vi "RT Driver VI.vi"(7 "Operation":T1, 11 "Device Reference in":T2 format="%.0x") -> (0 "Error Code":i32)   [LabVIEW 2016, in "PXImc Custom Device Engine.lvlib"]
uses:
  PXImc Custom Device Engine.lvlib
  <vilib>/NI Veristand/Custom Device API/Custom Device Item Ref.ctl
  <vilib>/NI Veristand/Custom Device API/Hardware Interface Driver VI Operation.ctl
  Shared/Compiled.Settings.ctl
  PXImc Router/Controls/Target Type.ctl
  PXImc Router/Controls/Router - Configuration.ctl
  PXImc Router/Controls/Router/Node Block R-W Properties.ctl
  PXImc Router/Controls/Router/Block Properties.ctl
  PXImc Router/Controls/Router/Router - PXImc Properties.ctl
  PXImc Router/Controls/Router/Router - PXImc Card Properties.ctl
  PXImc Router/Controls/Node Data.ctl
  PXImc Router/Controls/Node/Node - PXImc Parameters.ctl
  PXImc Router/Controls/Node/Node - Writer Data.ctl
  PXImc Router/Controls/Node/Node Ch Properties.ctl
  PXImc Router/Controls/Data Type.ctl
  PXImc Router/Controls/Node/Node - Readers Data.ctl
  PXImc Router/Controls/Node/Node - Reader Data.ctl
  RTStateVariables.ctl
  <vilib>/NI/NIVS Inline Async API/_VS Inline Async API/VS Inline Async API/VS Inline Async API.lvclass
  <vilib>/NI/NIVS Inline Async API/_VS Inline Async API/VS Inline Async API/VS Inline Async API.lvclass/VS Inline Async API.ctl
  <vilib>/NI/NIVS Inline Async API/_Data Access Engine/Data Access Engine/Data Access Engine.lvclass/Data Access Engine.ctl
  <vilib>/NI/NIVS Inline Async API/_Data Access Engine/Access Type Classes/Write/Write.lvclass/Write.ctl
  <vilib>/NI/NIVS Inline Async API/_Data Access Engine/Access Type Classes/ReadWrite/ReadWrite.lvclass/ReadWrite.ctl
  <vilib>/NI/NIVS Inline Async API/_Data Access Engine/Access Type Classes/Read/Read.lvclass/Read.ctl
  <vilib>/NI/NIVS Inline Async API/_Data Access Engine/Data Access Engine/Methods/Data.Engine.Read Data from HW.vi
  <vilib>/NI/NIVS Inline Async API/_VS Inline Async API/Error Handling Process/SubVIs/Error.GetError.vi
  <vilib>/NI/NIVS Inline Async API/_Data Access Engine/Data Access Engine/Methods/Data.Engine.Write Data to HW.vi
  <vilib>/NI/NIVS Inline Async API/_Data Access Engine/Access Type Classes/ReadWrite/ReadWrite.EngineData.vi
  <vilib>/NI/NIVS Inline Async API/_Data Access Engine/Access Type Classes/Write/Write.EngineData.vi
  <vilib>/NI/NIVS Inline Async API/_Data Access Engine/Access Type Classes/Read/Read.EngineData.vi
  <vilib>/NI Veristand/Custom Device API/NI VeriStand - Get Channel Value by Data Reference.vi
  <vilib>/NI Veristand/Custom Device API/NI VeriStand - Set Channel Value by Data Reference.vi
  <vilib>/NI Veristand/Custom Device API/NI VeriStand - Get Channel Values by Block Data Reference.vi
  Shared/Constants.vi
  <vilib>/NI Veristand/Custom Device API/Get Item Property (Variant).vi
  <vilib>/NI Veristand/Custom Device API/Global Data Refs.vi
  <vilib>/NI VeriStand/Custom Device API/Custom Device API.lvlib
  <vilib>/NI VeriStand/Custom Device Tools/Custom Device Utility Library/Custom Device Utility Library.lvlib
  Shared/PXImc Custom Device Shared.lvlib
  PXImc Router/PXImc Router.lvlib
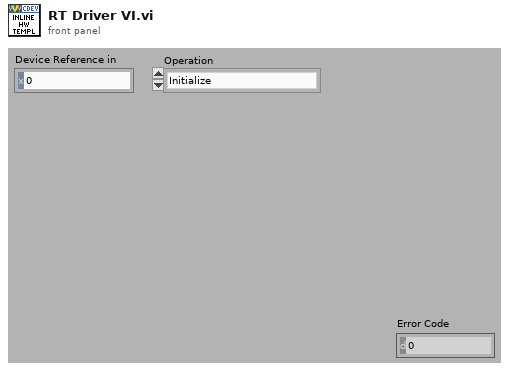
[diagram p1: front panel]
types:
  T1 = typedef "Custom Device API.lvlib/Hardware Interface Driver VI Operation.ctl" = enum16{"Initialize", "Start", "Read Data from HW", "Write Data to HW", "Close"}
  T2 = typedef "Custom Device API.lvlib/Custom Device Item Ref.ctl" = u64
  T3 = typedef "PXImc Custom Device Engine.lvlib/RTStateVariables.ctl" = cluster{"Async":refnum<class "VS Inline Async API.lvclass">, "Settings":T4}
  T4 = typedef "PXImc Custom Device Shared.lvlib/Compiled.Settings.ctl" = cluster{"Target Type":T5, "Router Properties":T6, "Node Data":T11, "Configuration Folder Path":path}
  T5 = typedef "PXImc Router.lvlib/Target Type.ctl" = enum16{"Router", "Node"}
  T6 = typedef "PXImc Router.lvlib/Router - Configuration.ctl" = cluster{"Target Type":T5, "Master Table Ref":refnum<data-value>, "Master Table Size (Bytes)":u32, "Node Properties":T7[], "Router - PXImc Properties":T9}
  T7 = typedef "PXImc Router.lvlib/Node Block R-W Properties.ctl" = cluster{"Node ID":u32, "# Reading Blocks":u32, "Node Writing Block":T8, "Node Reading Blocks":T8[]}
  T8 = typedef "PXImc Router.lvlib/Block Properties.ctl" = cluster{"Offset":u32, "Size (Bytes)":u32}
  T9 = typedef "PXImc Router.lvlib/Router - PXImc Properties.ctl" = cluster{"PXImc Cards Properties":T10[], "Connection Timeout (s)":dbl, "Readers Buffer Size":u64}
  T10 = typedef "PXImc Router.lvlib/Router - PXImc Card Properties.ctl" = cluster{"PXImc Resource Name":string, "Reader - PXImc Session Ref":refnum<k21>, "Writer - PXImc Session Ref":refnum<k21>, "Reader Conn ID":u16, "Writer Conn ID":u16}
  T11 = typedef "PXImc Router.lvlib/Node Data.ctl" = cluster{"Node Name":string, "PXImc Parameters":T12, "Local Data":T13, "Imported Data":T16}
  T12 = typedef "PXImc Router.lvlib/Node - PXImc Parameters.ctl" = cluster{"Resource Name":string, "Connection Timeout (s)":dbl, "Readers Buffer Size":u64, "Node PXImc Reader Conn Id":u16, "Node PXImc Writer Conn Id":u16, "Writer PXImc Session":refnum<k21>, "Reader PXImc Session":refnum<k21>}
  T13 = typedef "PXImc Router.lvlib/Node - Writer Data.ctl" = cluster{"Flattened Byte Buffer Ref":string, "Noder ID":u32, "Master Table Offest":u32, "Byte Buffer Size":u32, "Node Local Channels":T14[], "Node Local Channels Table":string[][]}
  T14 = typedef "PXImc Router.lvlib/Node Ch Properties.ctl" = cluster{"Name":string, "Value":dbl, "Data Type":T15}
  T15 = typedef "PXImc Router.lvlib/Data Type.ctl" = enum16{"Boolean", "SGL", "DBL", "I8", "I16", "I32", "I64", "U8", "U16", "U32", "U64"}
  T16 = typedef "PXImc Router.lvlib/Node - Readers Data.ctl" = cluster{"Flattened Byte Buffer Ref":string, "Byte Buffer Size":u64, "Readers Data Array":T17[], "Node Imported Channels Table":string[][]}
  T17 = typedef "PXImc Router.lvlib/Node - Reader Data.ctl" = cluster{"Noder ID":u32, "Master Table Offest":u32, "Byte Buffer Size":u64, "Node Imported Channels":T14[]}
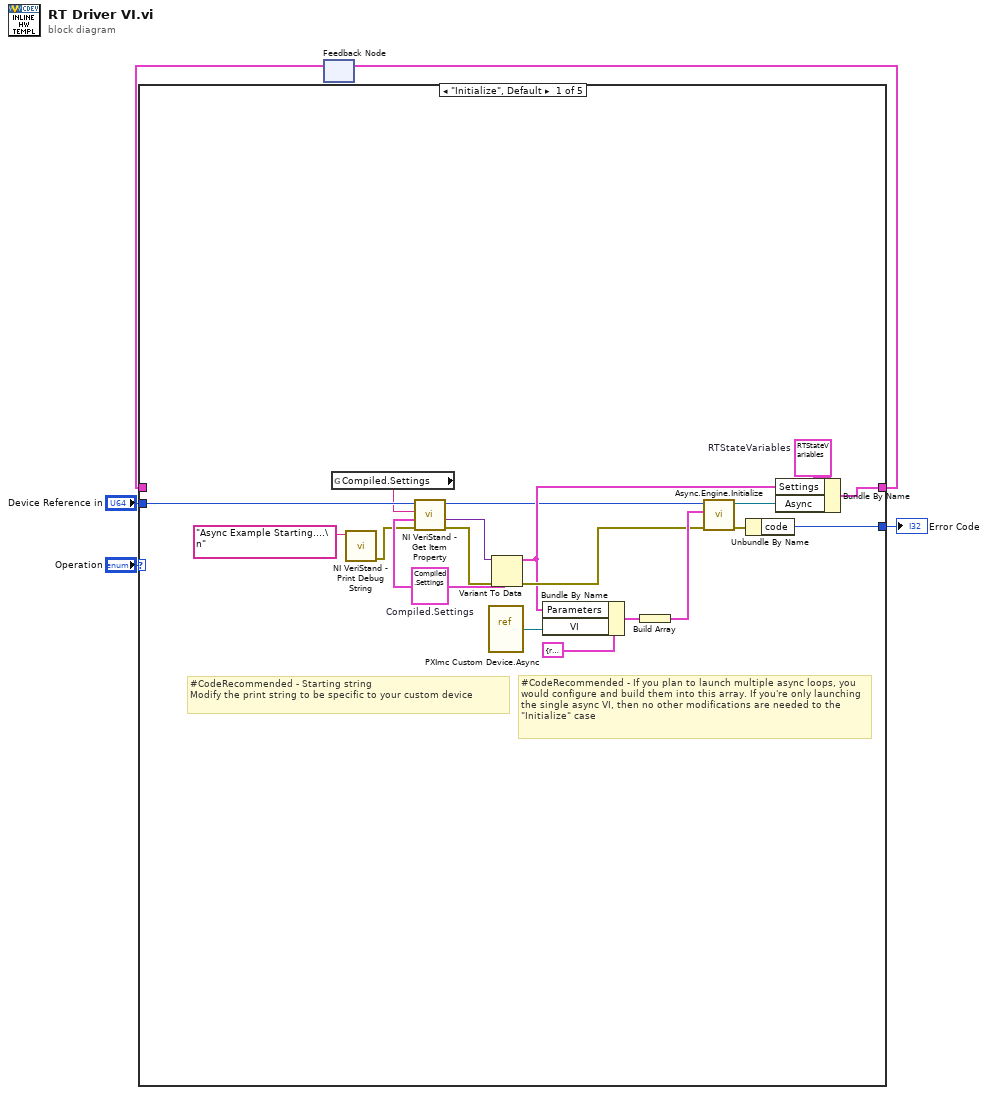
[diagram p0: block diagram]
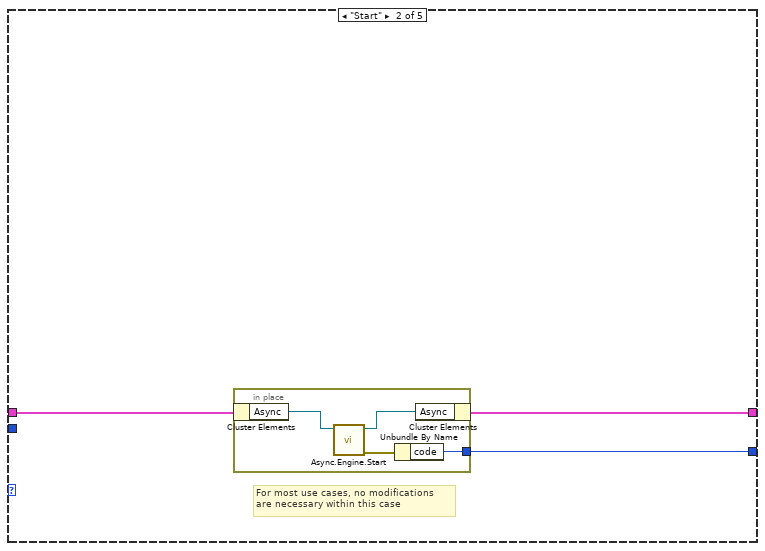
[diagram p2: hidden frame]
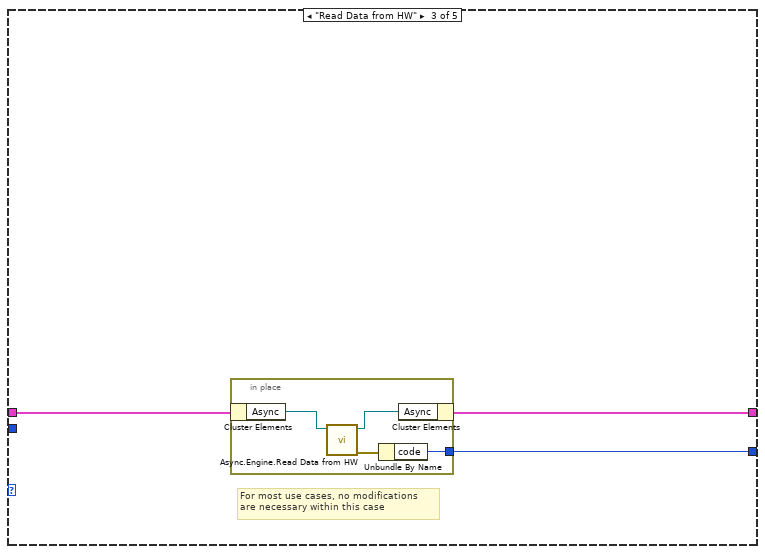
[diagram p3: hidden frame]
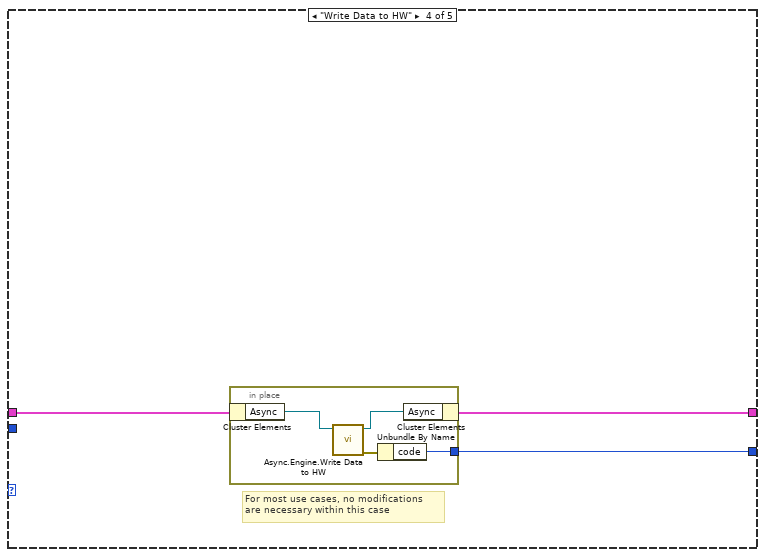
[diagram p4: hidden frame]
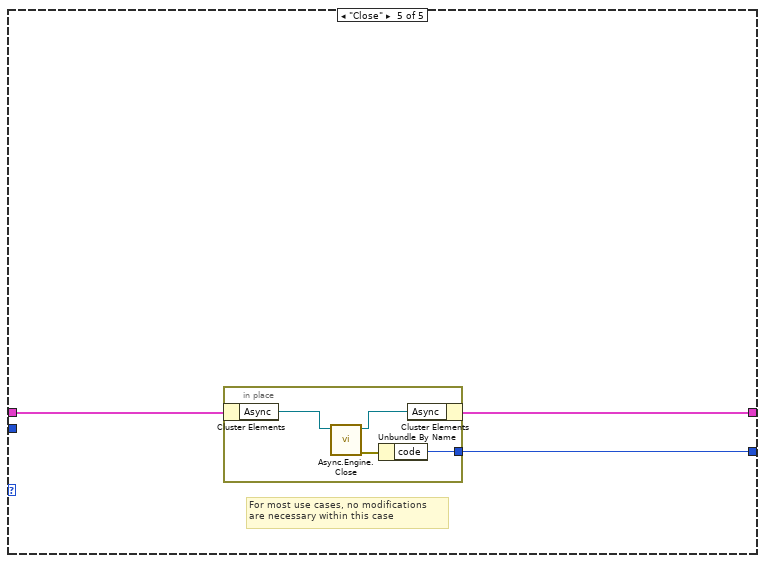
[diagram p5: hidden frame]
diagram:
  n1 = feedback #1() -> (w3:T3)  [unwired: 1 out]
  n2 = case shown="\"Initialize\", Default" "Operation" {
    tunnel: [w22 w26 w32 w39 w47] -> w4
    tunnel: w3 -> [_ w27 w34 w40 w48]
    tunnel: "Device Reference in" -> [w19 _ _ _ _]
    tunnel: [w24 w25 w33 w41 w46] -> w1
    frame "Initialize", Default {
      w15 = T3 {"Async"=refnum, "Settings"={"Target Type"=enum."Router", "Router Properties"={"Target Type"=enum."Router", "Master Table Ref"=refnum, "Master Table Size (Bytes)"=0, "Node Properties"=[], "Router - PXImc Properties"={"PXImc Cards Properties"=[], "Connection Timeout (s)"=0.0, "Readers Buffer Size"=0}}, "Node Data"={"Node Name"="", "PXImc Parameters"={"Resource Name"="", "Connection Timeout (s)"=0.0, "Readers Buffer Size"=0, "Node PXImc Reader Conn Id"=0, "Node PXImc Writer Conn Id"=0, "Writer PXImc Session"="", "Reader PXImc Session"=""}, "Local Data"={"Flattened Byte Buffer Ref"="", "Noder ID"=0, "Master Table Offest"=0, "Byte Buffer Size"=0, "Node Local Channels"=[], "Node Local Channels Table"=[]}, "Imported Data"={"Flattened Byte Buffer Ref"="", "Byte Buffer Size"=0, "Readers Data Array"=[], "Node Imported Channels Table"=[]}}, "Configuration Folder Path"=path ""}}  # RTStateVariables
      w16 = T4 {"Target Type"=enum."Router", "Router Properties"={"Target Type"=enum."Router", "Master Table Ref"=refnum, "Master Table Size (Bytes)"=0, "Node Properties"=[], "Router - PXImc Properties"={"PXImc Cards Properties"=[], "Connection Timeout (s)"=0.0, "Readers Buffer Size"=0}}, "Node Data"={"Node Name"="", "PXImc Parameters"={"Resource Name"="", "Connection Timeout (s)"=0.0, "Readers Buffer Size"=0, "Node PXImc Reader Conn Id"=0, "Node PXImc Writer Conn Id"=0, "Writer PXImc Session"="", "Reader PXImc Session"=""}, "Local Data"={"Flattened Byte Buffer Ref"="", "Noder ID"=0, "Master Table Offest"=0, "Byte Buffer Size"=0, "Node Local Channels"=[], "Node Local Channels Table"=[]}, "Imported Data"={"Flattened Byte Buffer Ref"="", "Byte Buffer Size"=0, "Readers Data Array"=[], "Node Imported Channels Table"=[]}}, "Configuration Folder Path"=path ""}  # Compiled.Settings
      # "#CodeRecommended - Starting string\nModify the print string to be specific to your custom device"
      # "#CodeRecommended - If you plan to launch multiple async loops, you would configure and build them into this array. If you're only launching the single async VI, then no other modifications are needed to the \"Initialize\" case"
      n3 = global read "Constants.vi" "Compiled.Settings"() -> (w17:string)
      n4 = call <vilib>:"NI VeriStand - Print Debug String.vi"("Message"="Async Example Starting....\n") -> ("error out"=w10:errorcluster)  [unwired: 10 in]
      n5 = call-poly <vilib>:"NI VeriStand - Get Item Property.vi"("error in (no error)"=w10, "Default Value"=w16, "Property Name"=w17, "Item Ref in"=w19) -> ("error out"=w6:errorcluster, "Value"=w18:variant, "Item Ref out"=w11:T2)  [unwired: 4 in, 1 out]
      n6 = vi-ref "PXImc Custom Device.Async.vi"() -> (w8:refnum<vi>)
      n7 = Variant To Data(error in=w6, type=w16, Variant=w18) -> (data=w12:T4, error out=w13:errorcluster)
      n8 = Bundle By Name(cluster=cluster{"VI":refnum<vi>, "Parameters":variant} {"VI"=refnum, "Parameters"=variant} ("Process"), "Parameters"=w12, "VI"=w8) -> (w20:cluster{"VI":refnum<vi>, "Parameters":variant})
      n9 = Build Array(w20) -> (w14:cluster{"VI":refnum<vi>, "Parameters":variant}[])
      n10 = call <vilib>:"Async.Engine.Initialize.vi"("error in (no error)"=w13, "Processes"=w14, "Custom Device Ref"=w11) -> ("error out"=w7:errorcluster, "Async"=w23:refnum<class "VS Inline Async API.lvclass">)  [unwired: 7 in]
      n11 = Unbundle By Name(w7) -> ("code"=w24:i32)
      n12 = Bundle By Name(cluster=w15, "Settings"=w12, "Async"=w23) -> (w22:T3)
    }
    frame "Start" {
      # "For most use cases, no modifications \nare necessary within this case"
      n13 = in-place {
        in-place-border: [w28] -> w25
        n14 = in-place-cluster #2(w27) -> ("Async"=w31:refnum<class "VS Inline Async API.lvclass">)
        n15 = call <vilib>:"Async.Engine.Start.vi"("VS Inline Async API in"=w31) -> ("error out"=w29:errorcluster, "VS Inline Async API out"=w30:refnum<class "VS Inline Async API.lvclass">)  [unwired: 9 in]
        n16 = Unbundle By Name(w29) -> ("code"=w28:i32)
        n17 = in-place-cluster #2("Async"=w30) -> (w26:T3)
      }
    }
    frame "Read Data from HW" {
      # "For most use cases, no modifications \nare necessary within this case"
      n18 = in-place {
        in-place-border: [w36] -> w33
        n19 = in-place-cluster #3(w34) -> ("Async"=w38:refnum<class "VS Inline Async API.lvclass">)
        n20 = call <vilib>:"Async.Engine.Read Data from HW.vi"("Async in"=w38) -> ("error out"=w35:errorcluster, "Async out"=w37:refnum<class "VS Inline Async API.lvclass">)  [unwired: 9 in]
        n21 = Unbundle By Name(w35) -> ("code"=w36:i32)
        n22 = in-place-cluster #3("Async"=w37) -> (w32:T3)
      }
    }
    frame "Write Data to HW" {
      # "For most use cases, no modifications \nare necessary within this case"
      n23 = in-place {
        in-place-border: [w45] -> w41
        n24 = in-place-cluster #4(w40) -> ("Async"=w43:refnum<class "VS Inline Async API.lvclass">)
        n25 = call <vilib>:"Async.Engine.Write Data to HW.vi"("VS Inline Async API in"=w43) -> ("error out"=w44:errorcluster, "VS Inline Async API out"=w42:refnum<class "VS Inline Async API.lvclass">)  [unwired: 9 in]
        n26 = Unbundle By Name(w44) -> ("code"=w45:i32)
        n27 = in-place-cluster #4("Async"=w42) -> (w39:T3)
      }
    }
    frame "Close" {
      # "For most use cases, no modifications \nare necessary within this case"
      n28 = in-place {
        in-place-border: [w50] -> w46
        n29 = in-place-cluster #5(w48) -> ("Async"=w52:refnum<class "VS Inline Async API.lvclass">)
        n30 = call <vilib>:"Async.Engine.Close.vi"("Async in"=w52) -> ("error out"=w49:errorcluster, "Async out"=w51:refnum<class "VS Inline Async API.lvclass">)  [unwired: 9 in]
        n31 = Unbundle By Name(w49) -> ("code"=w50:i32)
        n32 = in-place-cluster #5("Async"=w51) -> (w47:T3)
      }
    }
  }
  "Error Code" <- w1
  n33 = feedback-in #1(w4) -> ()
